vi "PH_Beckhoff_StepMot.Move and Stop.vi"(0 "AMS Net ID in":T1, 1 "ADS Error in":i32, 2 "Read and Write?":bool, 3 "# of Klemme [1, ...]":u32, 4 "Axis Activity in":T2 caption="Axis Activity", 5 "error in (no error)":errorcluster, 6 "Endswitch inverted?":bool, 7 "Move?":bool, 9 "Target":i32, 11 "Endswitch?":bool) -> (12 "Position":cluster{"Target":i32, "Current":i32}, 14 "AMS Net ID out":T1, 15 "ADS Error out":i32, 16 "Read and Write succesful?":bool, 17 "Status":T3, 18 "Axis Activity out":T2 caption="Axis Activity", 19 "error out":errorcluster)   [LabVIEW 2014, in "PH_Beckhoff_StepMot.lvlib"]
uses:
  PH_Beckhoff_StepMot.lvlib
  PH_Stepmotor_BaseClass/PH_Stepmotor_BaseClass.Axis Activity.ctl
  non_GPL/instr.lib/Beckhoff/Read and Write Data/Step Motor Klemmen/Beckhoff.Step Motor - Status.ctl
  non_GPL/instr.lib/Beckhoff/Read and Write Data/Step Motor Klemmen/Beckhoff.Step Motor - Status Byte.ctl
  non_GPL/instr.lib/Beckhoff/Read and Write Data/Step Motor Klemmen/Beckhoff.Step Motor - Status Word.ctl
  non_GPL/instr.lib/Beckhoff/Helpers/Beckhoff Access.ctl
  non_GPL/instr.lib/Beckhoff/Beckhoff - Driver np.lvlib
  PH_Stepmotor_BaseClass/PH_Stepmotor_BaseClass.lvlib
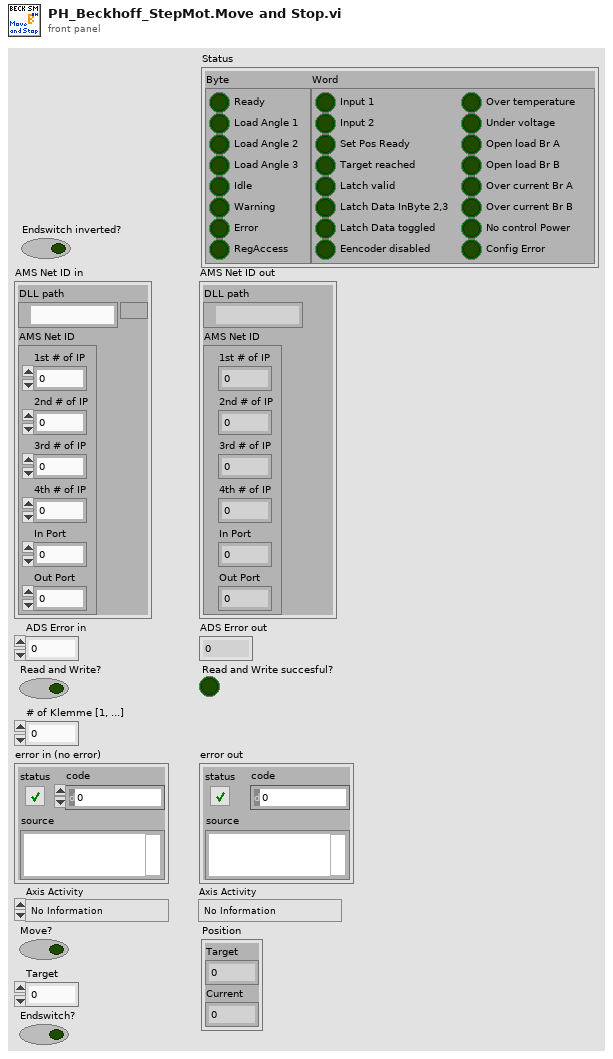
[diagram p1: front panel]
types:
  T1 = typedef "Beckhoff - Driver np.lvlib/Beckhoff Access.ctl" = cluster{"DLL path":path, "AMS Net ID":cluster{"1st # of IP":u8, "2nd # of IP":u8, "3rd # of IP":u8, "4th # of IP":u8, "In Port":u8, "Out Port":u8}}
  T2 = typedef "PH_Stepmotor_BaseClass.lvlib/PH_Stepmotor_BaseClass.Axis Activity.ctl" = enum16{"No Information", "stopped", "running", "Failure", "Alarm", "stopped at backward ES", "stopped at foreward ES"}
  T3 = typedef "Beckhoff - Driver np.lvlib/Beckhoff.Step Motor - Status.ctl" = cluster{"Byte":T4, "Word":T5}
  T4 = typedef "Beckhoff - Driver np.lvlib/Beckhoff.Step Motor - Status Byte.ctl" = cluster{"Ready":bool, "Load Angle 1":bool, "Load Angle 2":bool, "Load Angle 3":bool, "Idle":bool, "Warning":bool, "Error":bool, "RegAccess":bool}
  T5 = typedef "Beckhoff - Driver np.lvlib/Beckhoff.Step Motor - Status Word.ctl" = cluster{"Input 1":bool, "Input 2":bool, "Set Pos Ready":bool, "Target reached":bool, "Latch valid":bool, "Latch Data InByte 2,3":bool, "Latch Data toggled":bool, "Eencoder disabled":bool, "Over temperature":bool, "Under voltage":bool, "Open load Br A":bool, "Open load Br B":bool, "Over current Br A":bool, "Over current Br B":bool, "No control Power":bool, "Config Error":bool}
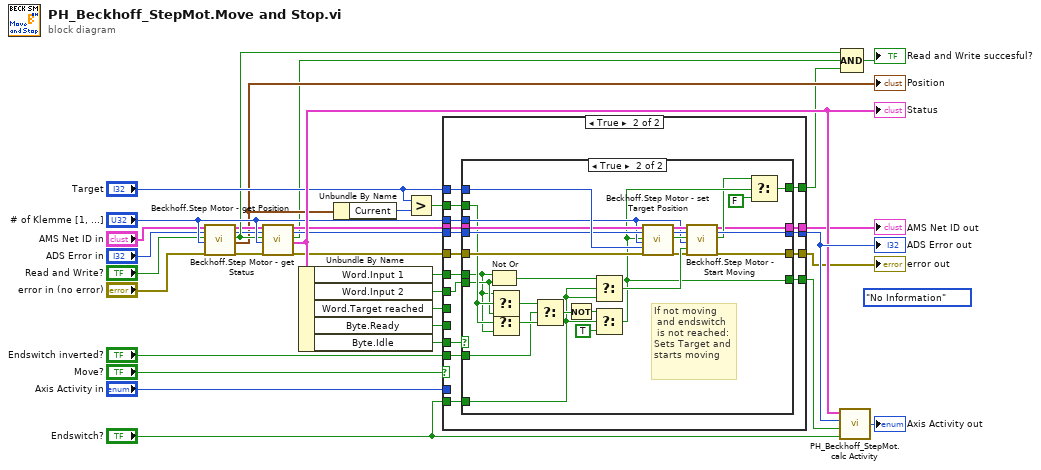
[diagram p0: block diagram]
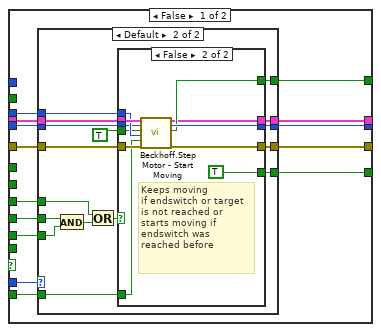
[diagram p2: hidden frame]
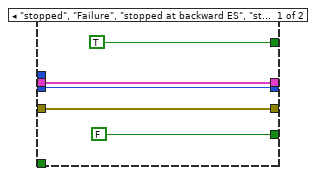
[diagram p3: hidden frame]
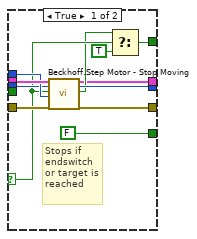
[diagram p4: hidden frame]
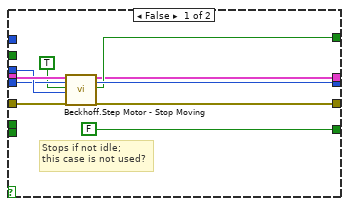
[diagram p5: hidden frame]
diagram:
  (unwired) PH_Stepmotor_BaseClass.Axis_Activity."No Information" ("Axis Activity in")
  n1 = call "Beckhoff.Step Motor - get Position.vi"("AMS Net ID in"="AMS Net ID in", "ADS Error in (0)"="ADS Error in", "Read?"="Read and Write?", "# of Klemme [1, ...]"="# of Klemme [1, ...]", "error in (no error)"="error in (no error)") -> ("AMS Net ID out"=w20:T1, "ADS Error out"=w21:i32, "Read successful?"=w22:bool, "Position"=w12:cluster{"Target":i32, "Current":i32}, "error out"=w23:errorcluster)  [unwired: 10 in]
  "Position" <- w12
  n2 = call "Beckhoff.Step Motor - get Status.vi"("AMS Net ID in"=w20, "ADS Error in (0)"=w21, "Read?"=w22, "# of Klemme [1, ...]"="# of Klemme [1, ...]", "error in (no error)"=w23) -> ("AMS Net ID out"=w17:T1, "ADS Error out"=w19:i32, "Read successful?"=w3:bool, "Status"=w31:T3, "error out"=w18:errorcluster)  [unwired: 10 in]
  "Status" <- w31
  n3 = Unbundle By Name(w31) -> ("Word.Input 1"=w8:bool, "Word.Input 2"=w9:bool, "Word.Target reached"=w26:bool, "Byte.Ready"=w27:bool, "Byte.Idle"=w10:bool)
  n4 = Unbundle By Name(w12) -> ("Current"=w11:i32)
  n5 = Greater?(x="Target", y=w11) -> (0:w7:bool)
  n6 = case shown="True" "Move?" {
    tunnel: "# of Klemme [1, ...]" -> [w48 w106]
    tunnel: "Target" -> [_ w108]
    tunnel: [w37 w107] -> w33
    tunnel: "Axis Activity in" -> [w38 _]
    tunnel: "Endswitch?" -> [w41 w105]
    tunnel: "Endswitch inverted?" -> [_ w104]
    tunnel: w10 -> [w42 w103]
    tunnel: w8 -> [_ w102]
    tunnel: w9 -> [_ w101]
    tunnel: w7 -> [_ w100]
    tunnel: w17 -> [w47 w99]
    tunnel: w18 -> [w45 w98]
    tunnel: [w39 w97] -> w28
    tunnel: w19 -> [w46 w96]
    tunnel: [w40 w95] -> w32
    tunnel: w26 -> [w44 _]
    tunnel: w27 -> [w43 _]
    tunnel: [w36 w94] -> w2
    tunnel: [w35 w93] -> w1
    frame False {
      n7 = case shown="Default" w38 {
        tunnel: w48 -> [_ w66]
        tunnel: [FALSE w69] -> w37
        tunnel: w41 -> [_ w56]
        tunnel: [w53 w67] -> w39
        tunnel: w45 -> [w53 w61]
        tunnel: w46 -> [w52 w62]
        tunnel: [w52 w64] -> w40
        tunnel: w47 -> [w49 w63]
        tunnel: w44 -> [_ w59]
        tunnel: w43 -> [_ w58]
        tunnel: w42 -> [_ w57]
        tunnel: [TRUE ("Write successful?") w55] -> w36
        tunnel: [w49 w54] -> w35
        frame "stopped", "Failure", "stopped at backward ES", "stopped at foreward ES" {
        }
        frame Default {
          n8 = And(x=w58, y=w57) -> (x .and. y?=w65:bool)
          n9 = Or(x=w59, y=w65) -> (x .or. y?=w68:bool)
          n10 = case shown="False" w68 {
            selector: w68 -> [w74 _]
            tunnel: w66 -> [w78 w88]
            tunnel: w56 -> [_ w89]
            tunnel: [FALSE TRUE] -> w69
            tunnel: w63 -> [w79 w92]
            tunnel: [w75 w90] -> w67
            tunnel: w61 -> [w80 w91]
            tunnel: w62 -> [w77 w86]
            tunnel: [w76 w87] -> w64
            tunnel: TRUE -> [_ w85]
            tunnel: [w72 w83] -> w55
            tunnel: [w70 w82] -> w54
            frame True {
              # "Stops if\nendswitch\nor target is\nreached"
              n11 = call "Beckhoff.Step Motor - Stop Moving.vi"("AMS Net ID in"=w79, "ADS Error in (0)"=w77, "Write?"=w74, "Klemme"=w78, "error in (no error)"=w80) -> ("AMS Net ID out"=w70:T1, "ADS Error out"=w76:i32, "Write successful?"=w73:bool, "error out"=w75:errorcluster)  [unwired: 11 in]
              n12 = Select(t=w73, s=w74, f=TRUE) -> (s? t:f=w72:bool)
            }
            frame False {
              # "Keeps moving\nif endswitch or target\nis not reached or\nstarts moving if\nendswitch was\nreached before"
              n13 = call "Beckhoff.Step Motor - Start Moving.vi"("AMS Net ID in"=w92, "ADS Error in (0)"=w86, "Write?"=w85, "Klemme"=w88, "End Switches enabled?"=w89, "error in (no error)"=w91) -> ("AMS Net ID out"=w82:T1, "ADS Error out"=w87:i32, "Write successful?"=w83:bool, "error out"=w90:errorcluster)  [unwired: 10 in]
            }
          }
        }
      }
    }
    frame True {
      n14 = case shown="True" w103 {
        tunnel: w108 -> [_ w145]
        tunnel: [FALSE w123] -> w107
        tunnel: w106 -> [w116 w131]
        tunnel: w105 -> [_ w130]
        tunnel: w104 -> [_ w124]
        tunnel: w102 -> [_ w126]
        tunnel: w101 -> [_ w127]
        tunnel: w100 -> [_ w128]
        tunnel: w99 -> [w117 w138]
        tunnel: w98 -> [w115 w139]
        tunnel: [w114 w140] -> w97
        tunnel: w96 -> [w113 w137]
        tunnel: [w111 w136] -> w95
        tunnel: [w110 w120] -> w94
        tunnel: [w109 w119] -> w93
        frame False {
          # "Stops if not idle;\nthis case is not used?"
          n15 = call "Beckhoff.Step Motor - Stop Moving.vi"("AMS Net ID in"=w117, "ADS Error in (0)"=w113, "Write?"=TRUE, "Klemme"=w116, "error in (no error)"=w115) -> ("AMS Net ID out"=w109:T1, "ADS Error out"=w111:i32, "Write successful?"=w110:bool, "error out"=w114:errorcluster)  [unwired: 11 in]
        }
        frame True {
          # "If not moving\n and endswitch\n is not reached:\nSets Target and\nstarts moving"
          n16 = Not Or(1:w127, 2:w126) -> (0:w143:bool)
          n17 = Select(t=w126, s=w128, f=w127) -> (s? t:f=w129:bool)
          n18 = Select(t=w127, s=w128, f=w126) -> (s? t:f=w125:bool)
          n19 = Select(t=w129, s=w124, f=w125) -> (s? t:f=w144:bool)
          n20 = Not(x=w144) -> (.not. x?=w142:bool)
          n21 = Select(t=w143, s=w130, f=w130) -> (s? t:f=w146:bool)
          n22 = Select(t=w142, s=w130, f=TRUE) -> (s? t:f=w123:bool)
          n23 = call "Beckhoff.Step Motor - set Target Position.vi"("AMS Net ID in"=w138, "ADS Error in (0)"=w137, "Write?"=w123, "# of Klemme [1, ...]"=w131, "Target Position"=w145, "error in (no error)"=w139) -> ("AMS Net ID out"=w135:T1, "ADS Error out"=w133:i32, "Write successful?"=w132:bool, "error out"=w134:errorcluster)  [unwired: 10 in]
          n24 = call "Beckhoff.Step Motor - Start Moving.vi"("AMS Net ID in"=w135, "ADS Error in (0)"=w133, "Write?"=w132, "Klemme"=w131, "End Switches enabled?"=w146, "error in (no error)"=w134) -> ("AMS Net ID out"=w119:T1, "ADS Error out"=w136:i32, "Write successful?"=w122:bool, "error out"=w140:errorcluster)  [unwired: 10 in]
          n25 = Select(t=w122, s=w123, f=FALSE) -> (s? t:f=w120:bool)
        }
      }
    }
  }
  "ADS Error out" <- w32
  "error out" <- w28
  "AMS Net ID out" <- w1
  n26 = call "PH_Beckhoff_StepMot.calc Activity.vi"("Endswitch?"="Endswitch?", "Moving"=w33, "ADS Error in"=w32, "Status"=w31) -> ("Axis Activity"=→"Axis Activity out":T2)
  n27 = Compound Arithmetic op=AND(w22, w3, w2) -> (→"Read and Write succesful?":bool)
